vi "Create.vi"(8 "error in (no error)":errorcluster, 10 "Size (Full)":cluster{"Width":u16, "Height":u16}, 11 "2D Picture":refnum<vi>) -> (0 "error out":errorcluster, 3 "Picture Control Canvas out":refnum<class "Picture Control Canvas.lvclass">)   [LabVIEW 2020, in "Glyph Drawer.lvlib" / "Picture Control Canvas.lvclass"]
uses:
  Picture Control Canvas.lvclass
  Picture Control Canvas.lvclass/Picture Control Canvas.ctl
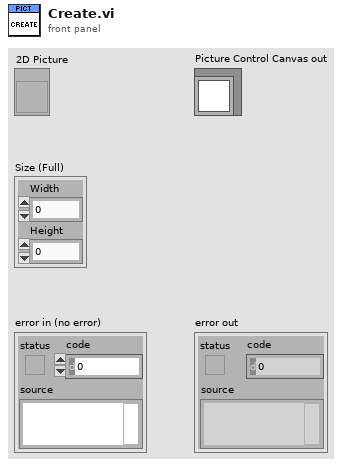
[diagram p1: front panel]
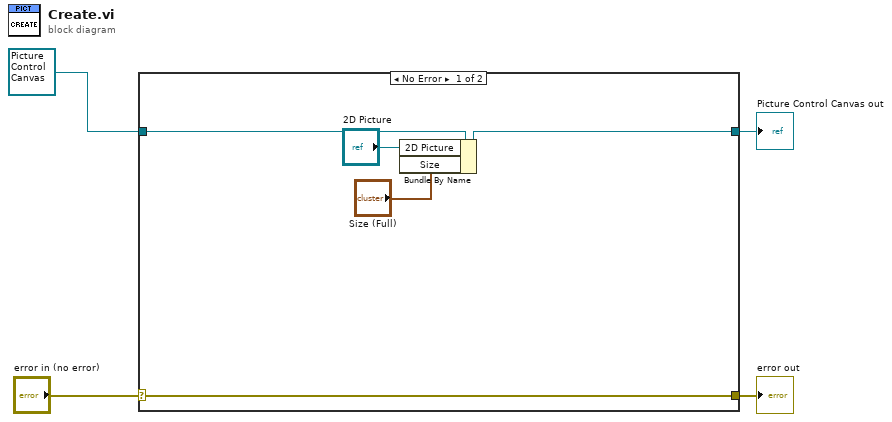
[diagram p0: block diagram]
diagram:
  n1 = case shown="No Error" "error in (no error)" {
    selector: "error in (no error)" -> [w8 w11]
    tunnel: [w8 w11] -> w3
    tunnel: [w7 w10] -> w1
    tunnel: refnum<class "Picture Control Canvas.lvclass"> refnum ("Picture Control Canvas in") -> [w9 w10]
    frame No Error {
      n2 = Bundle By Name(cluster=w9, "2D Picture"="2D Picture", "Size"="Size (Full)") -> (w7:refnum<class "Picture Control Canvas.lvclass">)
    }
    frame Error {
    }
  }
  "error out" <- w3
  "Picture Control Canvas out" <- w1
